vi "Trim Icon.vi"(4 "error in":errorcluster, 6 "subset rect":T1, 7 "Icon.lvclass in":refnum<class "Icon.lvclass">) -> (0 "error out":errorcluster, 3 "Icon.lvclass out":refnum<class "Icon.lvclass">)   [LabVIEW 2025, in "XNode Support.lvlib"]
uses:
  XNode Support.lvlib
  <vilib>/LabVIEW Icon API/lv_icon/Classes/Icon/Icon.lvclass
  <vilib>/LabVIEW Icon API/lv_icon/Classes/Layer/Layer.lvclass
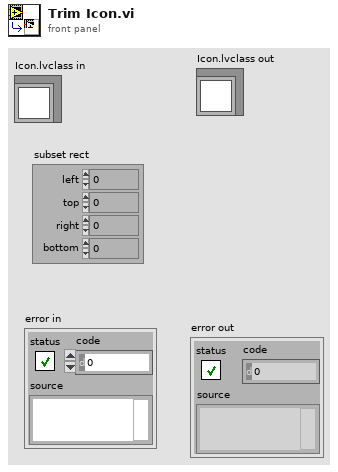
[diagram p1: front panel]
types:
  T1 = cluster{"left":i16, "top":i16, "right":i16, "bottom":i16}
  T2 = typedef "LVPoint32TypeDef.ctl" = cluster{"Horizontal":i32, "Vertical":i32}
  T3 = typedef "Layer.ctl" = cluster{"LayerIcon":picture, "LayerName":string, "Opacity":u8, "Visibility?":bool}
  T4 = typedef "imagedata.ctl" = cluster{"image type":i32, "image depth":i32, "image":u8[], "mask":u8[], "colors":u32[], "Rectangle":cluster{"left":i16, "top":i16, "right":i16, "bottom":i16}}
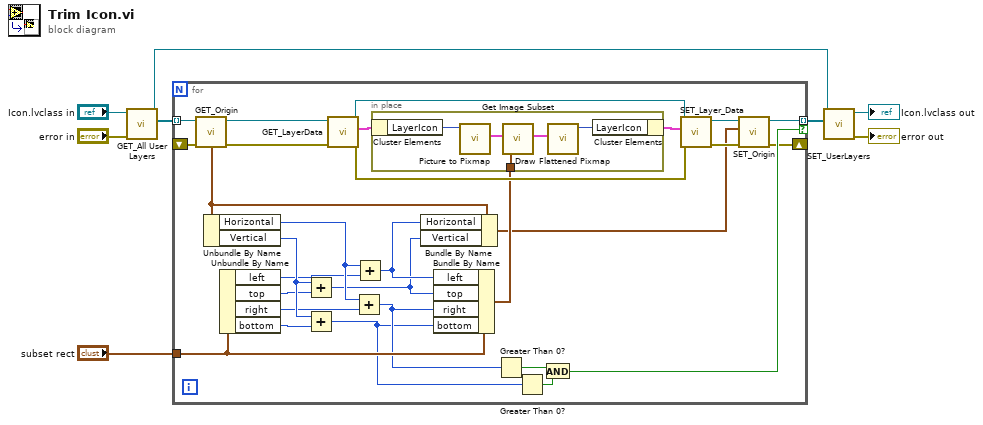
[diagram p0: block diagram]
diagram:
  n1 = call-dynamic "GET_All User Layers.vi"("error in (no error)"="error in", "Icon.lvclass in"="Icon.lvclass in") -> ("User Layer"=w4:refnum<class "Layer.lvclass">[], "Icon.lvclass out"=w5:refnum<class "Icon.lvclass">)  [unwired: 7 in, 1 out]
  n2 = for {
    tunnel: w4 -> [w32] mode=indexing
    tunnel: "subset rect" -> [w24]
    shift-right: [w19] -> _
    shift-left: _ -> [w33]
    tunnel: [w21] -> w3 mode=indexing if=w29
    n3 = call-dynamic "GET_Origin.vi"("error in (no error)"=w33, "Layer.lvclass in"=w32) -> ("error out"=w36:errorcluster, "Point32"=w18:T2, "Layer.lvclass out"=w37:refnum<class "Layer.lvclass">)  [unwired: 7 in]
    n4 = Unbundle By Name(w18) -> ("Horizontal"=w26:i32, "Vertical"=w25:i32)
    n5 = Unbundle By Name(w24) -> ("left"=w14:i16, "top"=w13:i16, "right"=w12:i16, "bottom"=w11:i16)
    n6 = Add(x=w25, y=w13) -> (x+y=w16:i32)
    n7 = Add(x=w25, y=w11) -> (x+y=w9:i32)
    n8 = call-dynamic "GET_LayerData.vi"("error in (no error)"=w36, "Layer.lvclass in"=w37) -> ("error out"=w34:errorcluster, "Data"=w28:T3, "Layer.lvclass out"=w35:refnum<class "Layer.lvclass">)  [unwired: 5 in, 2 out]
    n9 = Add(x=w26, y=w12) -> (x+y=w10:i32)
    n10 = Add(x=w26, y=w14) -> (x+y=w17:i32)
    n11 = Bundle By Name(cluster=w18, "Horizontal"=w17, "Vertical"=w16) -> (w15:T2)
    n12 = Bundle By Name(cluster=w24, "left"=w17, "top"=w16, "right"=w10, "bottom"=w9) -> (w23:T1)
    n13 = in-place {
      in-place-border: w23 -> [w40]
      n14 = in-place-cluster #1(w28) -> ("LayerIcon"=w39:picture)
      n15 = call <vilib>:"Picture to Pixmap.vi"("picture"=w39) -> ("image data"=w42:T4)  [unwired: 9 in, 1 out]
      n16 = call <vilib>:"Get Image Subset.vi"("subset rect"=w40, "image data"=w42) -> ("image subset"=w41:T4)  [unwired: 4 in, 1 out]
      n17 = call <vilib>:"Draw Flattened Pixmap.vi"("image data"=w41) -> ("new picture"=w38:picture)  [unwired: 8 in]
      n18 = in-place-cluster #1("LayerIcon"=w38) -> (w27:T3)
    }
    n19 = Greater Than 0?(x=w10) -> (x > 0?=w31:bool)
    n20 = Greater Than 0?(x=w9) -> (x > 0?=w30:bool)
    n21 = And(x=w31, y=w30) -> (x .and. y?=w29:bool)
    n22 = call-dynamic "SET_Layer_Data.vi"("error in (no error)"=w34, "Data"=w27, "Layer.lvclass in"=w35) -> ("error out"=w20:errorcluster, "Layer.lvclass out"=w22:refnum<class "Layer.lvclass">)  [unwired: 7 in]
    n23 = call-dynamic "SET_Origin.vi"("error in (no error)"=w20, "Point32"=w15, "Layer.lvclass in"=w22) -> ("error out"=w19:errorcluster, "Layer.lvclass out"=w21:refnum<class "Layer.lvclass">)  [unwired: 7 in]
  }
  n24 = call-dynamic "SET_UserLayers.vi"("Layers"=w3, "Icon.lvclass in"=w5) -> ("error out"=→"error out":errorcluster, "Icon.lvclass out"=→"Icon.lvclass out":refnum<class "Icon.lvclass">)  [unwired: 8 in]
